vi "Write Pin.vi"(0 "Arduino in":refnum<class "Arduino.lvclass">, 5 "Port":dbl, 7 "Pin":dbl, 9 "Value":bool, 11 "error in (no error)":errorcluster) -> (4 "Arduino out":refnum<class "Arduino.lvclass">, 15 "error out":errorcluster)   [LabVIEW 2020, in "Arduino.lvclass"]
doc: "Write Pin es el vi donde se escribe el valor del puerto en binario para que sea recibido por el microcontrolador y pueda encender o apagar el led correspondiente"
uses:
  Arduino.lvclass
  Arduino.lvclass/Arduino.ctl
  a9d43991-ca51-4a58-bcd7-32ef1cbfca89.vi
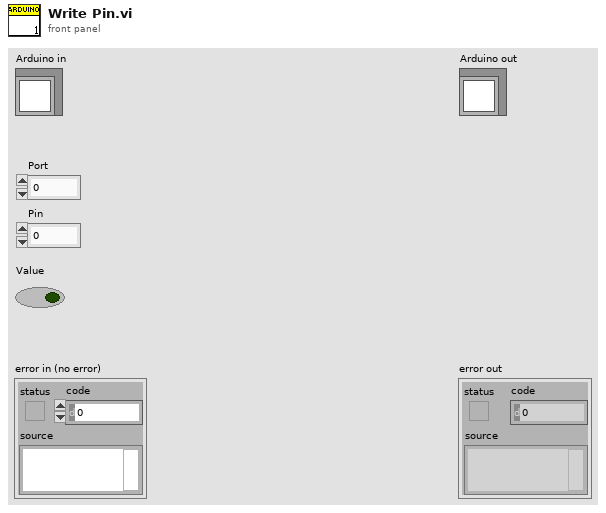
[diagram p1: front panel]
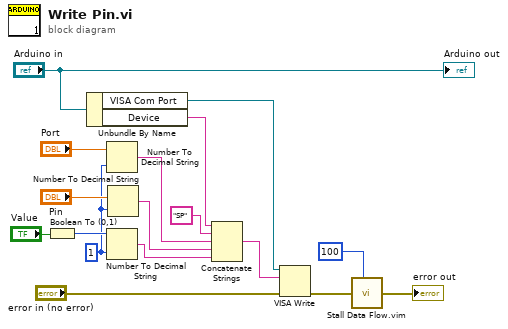
[diagram p0: block diagram]
diagram:
  w3 = i16 1 ("width (-)")
  n1 = Boolean To (0,1)(Boolean="Value") -> (0, 1=w6:i16)
  n2 = Unbundle By Name("Arduino in") -> ("VISA Com Port"=w14:refnum<visa-resource-name>, "Device"=w12:string)
  n3 = Number To Decimal String(number="Port", width (-)=w3) -> (decimal integer string=w10:string)
  n4 = Number To Decimal String(number=w6, width (-)=w3) -> (decimal integer string=w5:string)
  n5 = Number To Decimal String(number="Pin", width (-)=w3) -> (decimal integer string=w4:string)
  n6 = Concatenate Strings(w12, "SP" ("string"), w10, w4, w5) -> (w13:string)
  n7 = VISA Write(VISA resource name=w14, write buffer=w13, error in (no error)="error in (no error)") -> (error out=w15:errorcluster)  [unwired: 2 out]
  n8 = call "Stall Data Flow.vim"("value in"=w15, "milliseconds to wait"=u32 100) -> ("value out"=→"error out":errorcluster)  [unwired: 1 out]
  "Arduino out" <- "Arduino in"
